vi "Decode Remaining Length.vi"(11 "Packet w/o 1st byte":u8[](array[numeric]) format="%08b") -> (1 "Malformed Remaining Length":bool, 2 "Remaining Length (bytes)":u32, 3 "Remaining Packet":u8[](array[numeric]) format="%08b")   [LabVIEW 2013, in "MQTT_Control_Packets.lvlib" / "ControlPacket.lvclass"]
uses:
  ControlPacket.lvclass
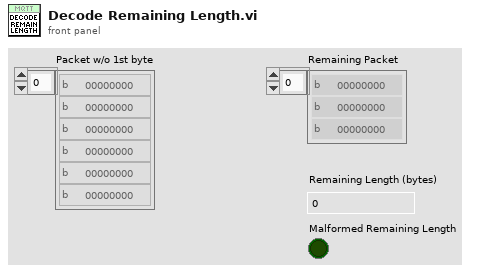
[diagram p1: front panel]
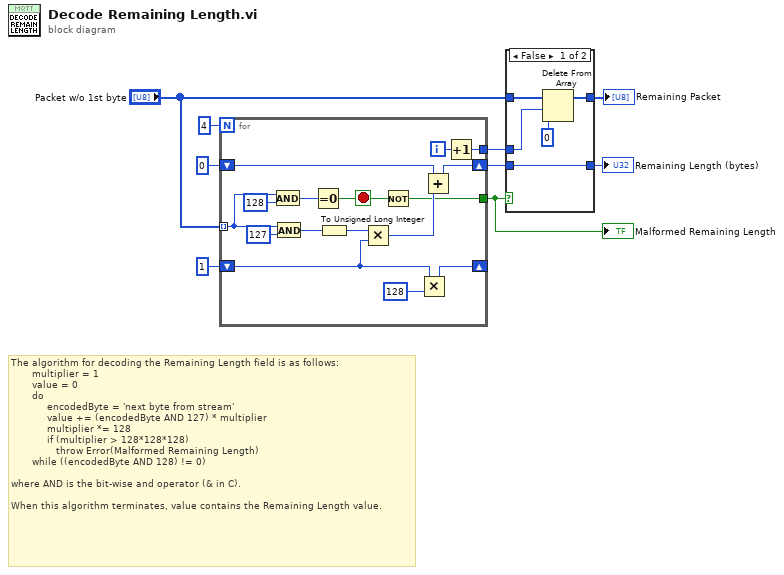
[diagram p0: block diagram]
diagram:
  # "The algorithm for decoding the Remaining Length field is as follows:\n       multiplier = 1\n       value = 0\n       do\n            encodedByte = 'next byte from stream'\n            value += (encodedByte AND 127) * multiplier\n            multiplier *= 128\n            if (multiplier > 128*128*128)\n               throw Error(Malformed Remaining Length)\n       while ((encodedByte AND 128) != 0)\n\nwhere AND is the bit-wise and operator (& in C).\n\nWhen this algorithm terminates, value contains the Remaining Length value."
  n1 = for {
    N: 4 -> [_]
    tunnel: "Packet w/o 1st byte" -> [w15] mode=indexing
    shift-right: [w24] -> _
    shift-left: u32 1 -> [w19]
    shift-right: [w23] -> w5
    shift-left: u32 0 -> [w22]
    tunnel: [w12] -> w6
    tunnel: [w10] -> w3
    i -> [w11]
    stop <- w13 stop-if-true
    n2 = And(x=w15, y=u8 128) -> (x .and. y?=w14:u8)
    n3 = And(x=w15, y=u8 127) -> (x .and. y?=w20:u8)
    n4 = Equal To 0?(x=w14) -> (x = 0?=w13:bool)
    n5 = To Unsigned Long Integer(number=w20) -> (unsigned 32bit integer=w18:u32)
    n6 = Multiply(x=w18, y=w19) -> (x*y=w16:u32)
    n7 = Not(x=w13) -> (.not. x?=w12:bool)
    n8 = Multiply(x=w19, y=u32 128) -> (x*y=w24:u32)
    n9 = Add(x=w22, y=w16) -> (x+y=w23:u32)
    n10 = Increment(x=w11) -> (x+1=w10:i32)
  }
  "Malformed Remaining Length" <- w6
  n11 = case shown="False" w6 {
    tunnel: "Packet w/o 1st byte" -> [w30 w31]
    tunnel: [w29 w31] -> w2
    tunnel: w5 -> [w28 _]
    tunnel: [w28 _] -> w4
    tunnel: w3 -> [w27 _]
    frame False {
      n12 = Delete From Array(array=w30, length=w27, index=0) -> (array with subset deleted=w29:u8[])  [unwired: 1 out]
    }
    frame True {
    }
  }
  "Remaining Length (bytes)" <- w4
  "Remaining Packet" <- w2
